vi "Inspect.vi"(6 "Listened To Msg":bool, 9 "Msg in":refnum<class "Msg.lvclass">, 10 "Within Msg Set":bool, 11 "Core Actor in":refnum<class "Core Actor.lvclass">) -> (1 "Msg out":refnum<class "Msg.lvclass">, 3 "Core Actor out":refnum<class "Core Actor.lvclass">)   [LabVIEW 2025, in "jettl.lvlib" / "Core Actor.lvlib" / "Core Actor.lvclass"]
uses:
  Core Actor.lvclass
  Msg/Msg.lvclass
  Core Actor.lvclass/Core Actor.ctl
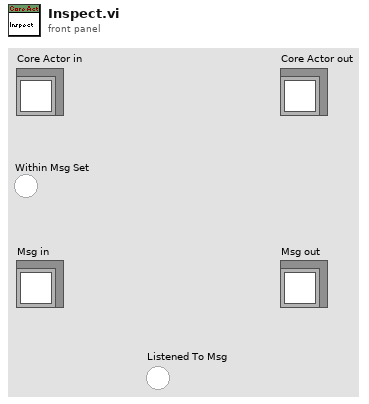
[diagram p1: front panel]
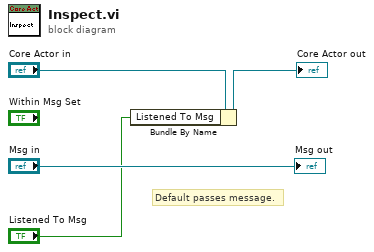
[diagram p0: block diagram]
diagram:
  # "Default passes message."
  n1 = Bundle By Name(cluster="Core Actor in", "Listened To Msg"="Listened To Msg") -> (→"Core Actor out":refnum<class "Core Actor.lvclass">)
  "Msg out" <- "Msg in"
